vi "doAction.vi"(8 "error in (no error)":errorcluster, 10 "ContextData In":refnum<class "ContextData.lvclass">, 11 "Wait Event in":refnum<class "Wait Event.lvclass">) -> (0 "error out":errorcluster, 2 "ContextData Out":refnum<class "ContextData.lvclass">, 3 "Wait Event out":refnum<class "Wait Event.lvclass">)   [LabVIEW 2019, in "Wait Event.lvclass"]
uses:
  Wait Event.lvclass
  ContextData/ContextData.lvclass
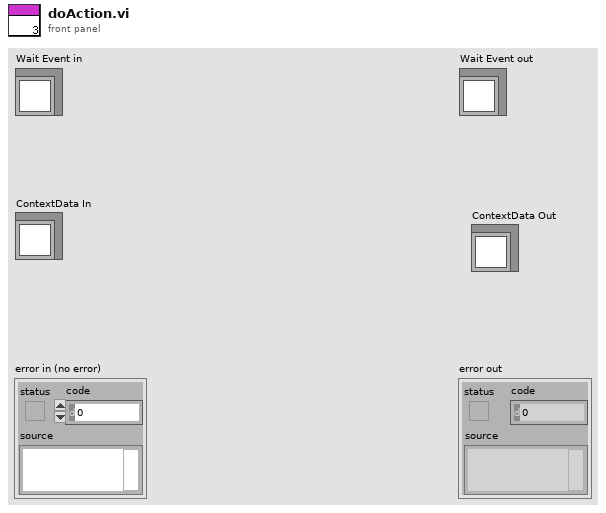
[diagram p1: front panel]
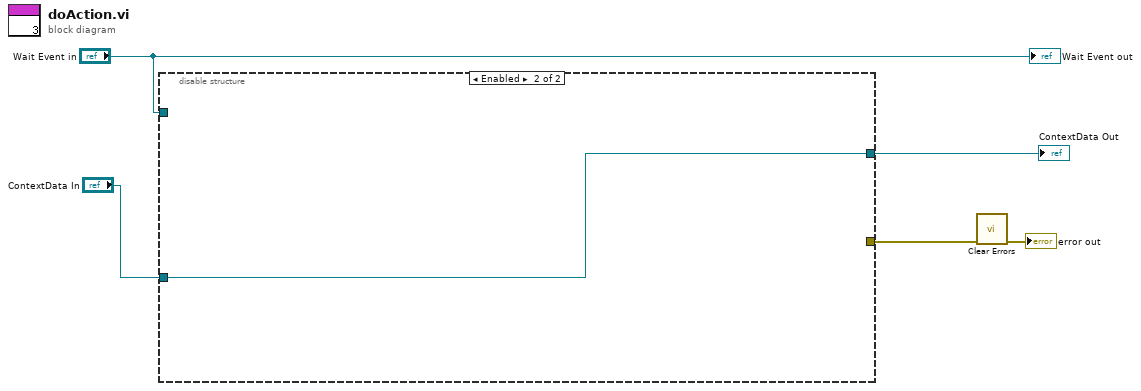
[diagram p0: block diagram]
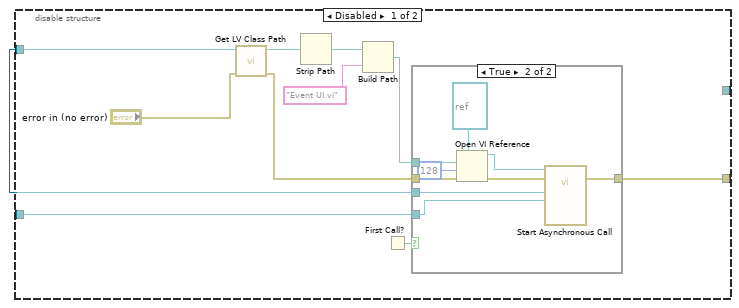
[diagram p2: hidden frame]
diagram:
  n1 = disable-structure shown="Enabled" {
    disable-tunnel: "Wait Event in" -> [w9 _]
    disable-tunnel: [w8 _] -> w3
    disable-tunnel: "ContextData In" -> [w6 w26]
    disable-tunnel: [_ w26] -> w1
    frame Disabled {
      n2 = call <vilib>:"Get LV Class Path.vi"("error in (no error)"="error in (no error)", "object"=w9) -> ("error out"=w13:errorcluster, "class path"=w15:path)  [unwired: 8 in]
      n3 = Strip Path(path=w15) -> (stripped path=w10:path)  [unwired: 1 out]
      n4 = Build Path(base path=w10, name or relative path="Event UI.vi") -> (appended path=w11:path)
      n5 = First Call?() -> (First Call?: T/F=w7:bool)
      n6 = case shown="True" w7 {
        tunnel: w13 -> [w16 w25]
        tunnel: w11 -> [_ w24]
        tunnel: w9 -> [_ w23]
        tunnel: [w16 w20] -> w8
        tunnel: w6 -> [_ w17]
        frame False {
        }
        frame True {
          n7 = Open VI Reference(type specifier VI Refnum (for type only)=refnum<vi> refnum, vi path=w24, options=128, error in (no error)=w25) -> (vi reference=w19:refnum<vi>, error out=w22:errorcluster)  [unwired: 2 in]
          n8 = call-by-ref "Start Asynchronous Call"(reference=w19, error in=w22, "ContextData In"=w17, "Wait Event in"=w23) -> (error out=w20:errorcluster)  [unwired: 8 in, 3 out]
        }
      }
    }
    frame Enabled {
    }
  }
  "ContextData Out" <- w1
  n9 = call <vilib>:"Clear Errors.vi"("error in (no error)"=w3) -> ("error out"=→"error out":errorcluster)  [unwired: 5 in, 1 out]
  "Wait Event out" <- "Wait Event in"
